vi "Simulator SNA Complex Resample (Single Shot Linear Interpolation).vi"(6 "#elements":i32, 8 "error in":errorcluster, 9 "t0":timestamp format="%<%.4X>T", 10 "dt":dbl=1.0 format="%.2p", 11 "waveform in":waveform(cdb)) -> (0 "error out":errorcluster, 3 "resampled waveform out":waveform(cdb))   [LabVIEW 2011]
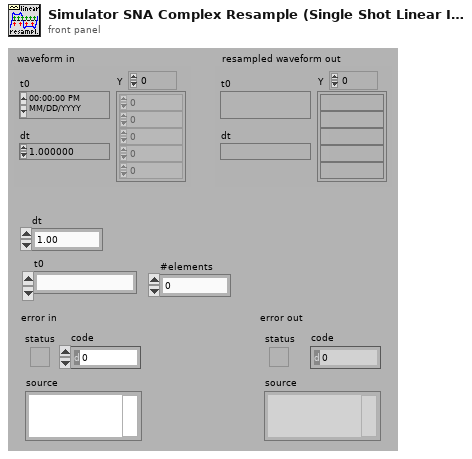
[diagram p1: front panel]
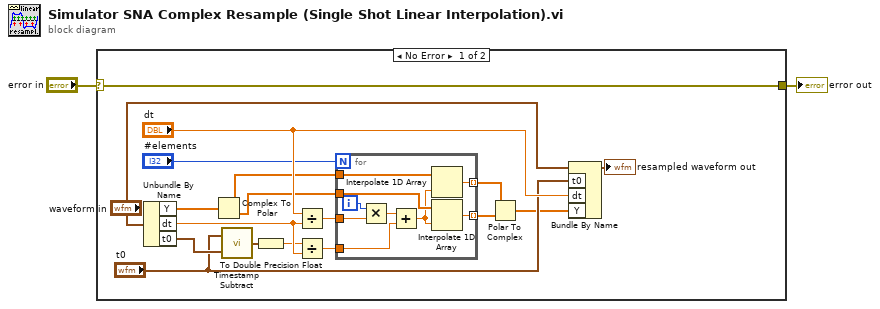
[diagram p0: block diagram]
diagram:
  n1 = case shown="No Error" "error in" {
    selector: "error in" -> [w13 w30]
    tunnel: [w13 w30] -> w1
    frame No Error {
      n2 = Unbundle By Name("waveform in") -> ("Y"=w8:cdb[], "dt"=w15:dbl, "t0"=w12:timestamp)
      n3 = Complex To Polar(r * e^(i*theta)=w8) -> (r=w7:dbl[], theta=w6:dbl[])
      n4 = call <vilib>:"Timestamp Subtract.vi"("y"=w12, "x"="t0") -> ("x - y"=w9:timestamp)
      n5 = To Double Precision Float(number=w9) -> (double precision float=w10:dbl)
      n6 = Divide(x="dt", y=w15) -> (x/y=w18:dbl)
      n7 = Divide(x=w10, y=w15) -> (x/y=w17:dbl)
      n8 = for {
        N: "#elements" -> [_]
        tunnel: w18 -> [w28]
        tunnel: w7 -> [w25]
        tunnel: [w22] -> w4 mode=indexing
        tunnel: w17 -> [w26]
        tunnel: w6 -> [w24]
        tunnel: [w21] -> w5 mode=indexing
        i -> [w29]
        n9 = Multiply(x=w29, y=w28) -> (x*y=w27:dbl)
        n10 = Add(x=w27, y=w26) -> (x+y=w23:dbl)
        n11 = Interpolate 1D Array(1:w23, 2:w25) -> (0:w21:dbl)
        n12 = Interpolate 1D Array(1:w23, 2:w24) -> (0:w22:dbl)
      }
      n13 = Polar To Complex(1:w4, 2:w5) -> (0:w3:cdb[])
      n14 = Bundle By Name(cluster="waveform in", "t0"="t0", "dt"="dt", "Y"=w3) -> (→"resampled waveform out":waveform(cdb))
    }
    frame Error {
    }
  }
  "error out" <- w1
